vi "Write Variant Data.vi"(8 "error in (no error)":errorcluster, 10 "data":variant, 11 "Base in":refnum<class "Base.lvclass">) -> (0 "error out":errorcluster, 3 "Base out":refnum<class "Base.lvclass">)   [LabVIEW 2020, in "PV Access.lvlib" / "PV Data.lvlib" / "Base.lvclass"]
uses:
  Base.lvclass
  Base.lvclass/Base.ctl
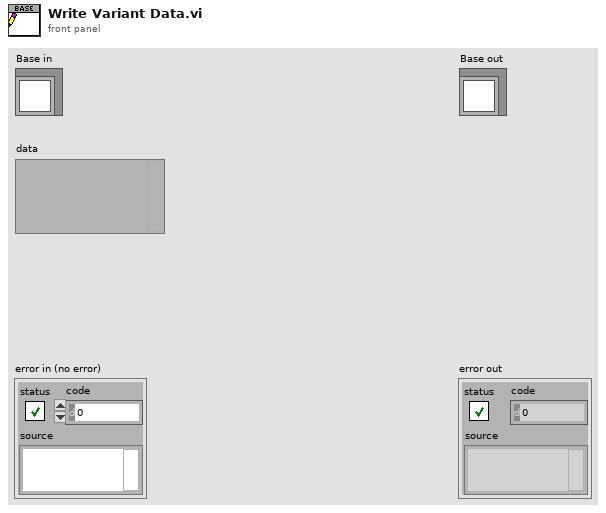
[diagram p1: front panel]
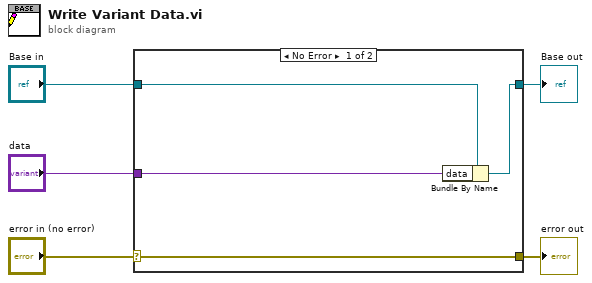
[diagram p0: block diagram]
diagram:
  n1 = case shown="No Error" "error in (no error)" {
    selector: "error in (no error)" -> [w9 w10]
    tunnel: [w9 w10] -> w4
    tunnel: [w7 w11] -> w2
    tunnel: "Base in" -> [w8 w11]
    tunnel: "data" -> [w6 _]
    frame No Error {
      n2 = Bundle By Name(cluster=w8, "data"=w6) -> (w7:refnum<class "Base.lvclass">)
    }
    frame Error {
    }
  }
  "error out" <- w4
  "Base out" <- w2
